vi "SCPI Query.vi"(8 "error in (no error)":errorcluster, 9 "byte count":u32=512, 10 "SCPI QUERY":string, 11 "36234A in":refnum<class "36234A.lvclass">) -> (0 "error out":errorcluster, 2 "read buffer":string, 3 "36234A out":refnum<class "36234A.lvclass">)   [LabVIEW 2019, in "36234A.lvlib" / "36234A.lvclass"]
uses:
  Library/36234A.lvclass
  Library/36234A.lvclass/36234A.ctl
  <instrlib>/Keysight E36000 Series/Keysight E36000 Series.lvlib
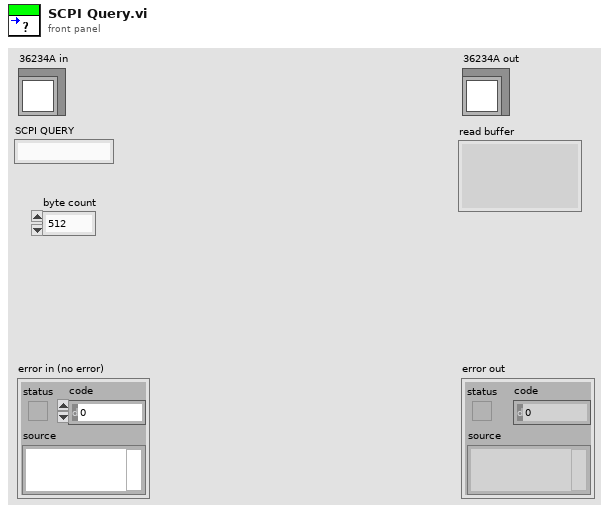
[diagram p1: front panel]
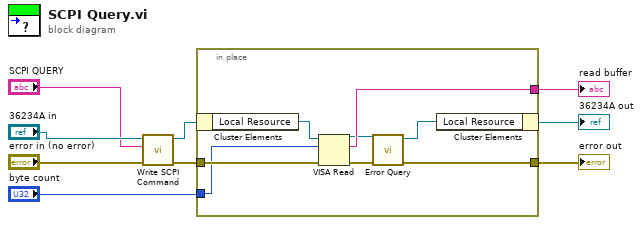
[diagram p0: block diagram]
diagram:
  n1 = call "Write SCPI Command.vi"("error in (no error)"="error in (no error)", "SCPI Command"="SCPI QUERY", "36234A in"="36234A in") -> ("error out"=w4:errorcluster, "36234A out"=w6:refnum<class "36234A.lvclass">)  [unwired: 7 in]
  n2 = in-place {
    in-place-border: w4 -> [w16]
    in-place-border: [w11] -> w3
    in-place-border: [w15] -> w2
    in-place-border: "byte count" -> [w14]
    n3 = in-place-cluster #1(w6) -> ("Local Resource"=w17:refnum<visa-resource-name>)
    n4 = VISA Read(VISA resource name=w17, byte count=w14, error in (no error)=w16) -> (VISA resource name out=w13:refnum<visa-resource-name>, read buffer=w15:string, error out=w12:errorcluster)  [unwired: 1 out]
    n5 = call <instrlib>:"Error Query.vi"("error in (no error)"=w12, "VISA resource name"=w13) -> ("error out"=w11:errorcluster, "VISA resource name out"=w10:refnum<visa-resource-name>)  [unwired: 6 in, 2 out]
    n6 = in-place-cluster #1("Local Resource"=w10) -> (→"36234A out":refnum<class "36234A.lvclass">)
  }
  "error out" <- w3
  "read buffer" <- w2
